vi "Start.vi"(4 "Creator":refnum<user-event>, 6 "Creator Alias":string, 7 "Path":path, 8 "Self Alias":string, 9 "Queue of Init":refnum<queue>, 10 "Actor":refnum<class "Actor.lvclass">) -> (0 "error out":errorcluster)   [LabVIEW 2021, in "jettl.lvlib" / "Temporary Actor.lvlib" / "jettl Actor.lvclass"]
uses:
  jettl Actor.lvclass
  Actor/Actor.lvclass
  Msg/Msg.lvclass
  Init.ctl
  jettl.vi
  jettl Actor.lvclass/jettl Actor.ctl
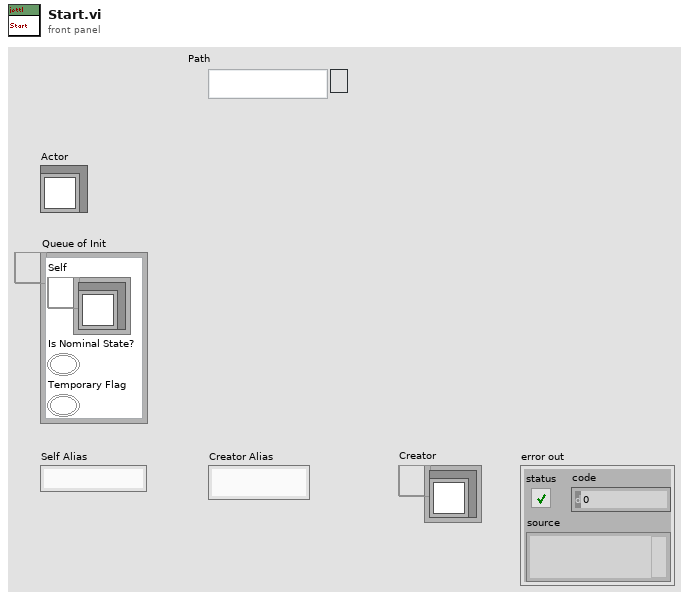
[diagram p1: front panel]
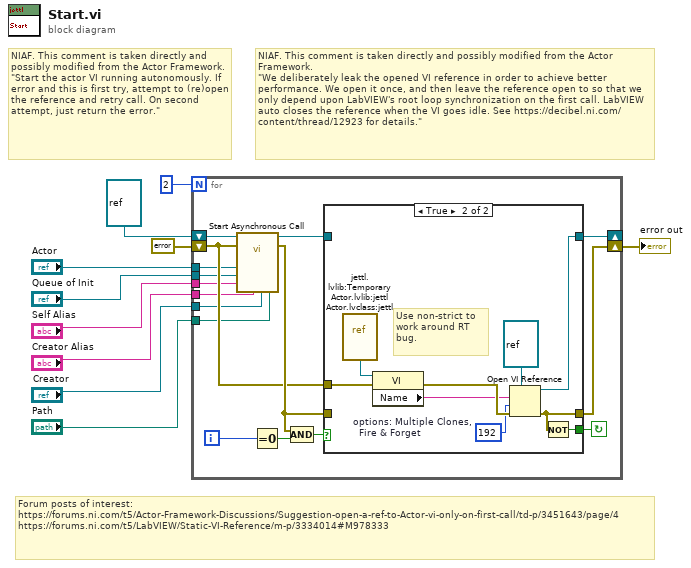
[diagram p0: block diagram]
diagram:
  # "Forum posts of interest:\nhttps://forums.ni.com/t5/Actor-Framework-Discussions/Suggestion-open-a-ref-to-Actor-vi-only-on-first-call/td-p/3451643/page/4\nhttps://forums.ni.com/t5/LabVIEW/Static-VI-Reference/m-p/3334014#M978333"
  # "NIAF. This comment is taken directly and possibly modified from the Actor Framework.\n\"We deliberately leak the opened VI reference in order to achieve better performance. We open it once, and then leave the reference open to so that we only depend upon LabVIEW's root loop synchronization on the first call. LabVIEW auto closes the reference when the VI goes idle. See https://decibel.ni.com/content/thread/12923 for details.\""
  # "NIAF. This comment is taken directly and possibly modified from the Actor Framework.\n\"Start the actor VI running autonomously. If error and this is first try, attempt to (re)open the reference and retry call. On second attempt, just return the error.\""
  n1 = for {
    N: 2 -> [_]
    shift-right: [w26] -> _
    shift-left: refnum<vi> refnum -> [w25]
    shift-right: [w23] -> w8
    shift-left: errorcluster {"status"=FALSE, "code"=0, "source"=""} ("error out") -> [w17]
    tunnel: "Actor" -> [w16]
    tunnel: "Self Alias" -> [w15]
    tunnel: "Creator Alias" -> [w14]
    tunnel: "Queue of Init" -> [w13]
    tunnel: "Creator" -> [w12]
    tunnel: "Path" -> [w11]
    i -> [w20]
    stop <- w18 continue-if-true
    n2 = call-by-ref "Start Asynchronous Call"(reference=w25, error in=w17, "Path"=w11, "Creator"=w12, "Creator Alias"=w14, "Self Alias"=w15, "Queue of Init"=w13, "jettl"=w16) -> (reference out=w24:refnum<vi>, error out=w19:errorcluster)  [unwired: 6 in]
    n3 = Equal To 0?(x=w20) -> (x = 0?=w21:bool)
    n4 = Compound Arithmetic op=AND(w19, w21) -> (w22:bool)
    n5 = case shown="True" w22 {
      tunnel: [w28 w34] -> w26
      tunnel: [w27 w32] -> w23
      tunnel: w24 -> [w28 _]
      tunnel: w19 -> [w27 _]
      tunnel: [_ w33] -> w18
      tunnel: w17 -> [_ w31]
      frame False {
      }
      frame True {
        w35 = 192  # options: Multiple Clones,   Fire & Forget
        # "Use non-strict to work around RT bug."
        n6 = vi-ref "jettl.lvlib:Temporary Actor.lvlib:jettl Actor.lvclass:jettl.vi"() -> (w30:refnum<vi>)
        n7 = property class="VI"(reference=w30, error in=w31) -> (error out=w37:errorcluster, "Name"=w36:string)  [unwired: 1 out]
        n8 = Open VI Reference(type specifier VI Refnum (for type only)=refnum<vi> refnum, vi path=w36, options=w35, error in (no error)=w37) -> (vi reference=w34:refnum<vi>, error out=w32:errorcluster)  [unwired: 2 in]
        n9 = Not(x=w32) -> (.not. x?=w33:bool)
      }
    }
  }
  "error out" <- w8
